vi "Construct.vi"(8 "series":i32(ring)=2 items=["DVP", "AS"], 9 "port":i32=502, 10 "station":u8=1, 11 "ipAddress":string="192.168.1.88") -> (3 "MelsecMcNet out":refnum<class "DeltaTcp.lvclass">)   [LabVIEW 2020, in "HslCommunication.lvlib" / "DeltaTcp.lvclass"]
uses:
  DeltaTcp.lvclass
  DeltaTcp.lvclass/DeltaTcp.ctl
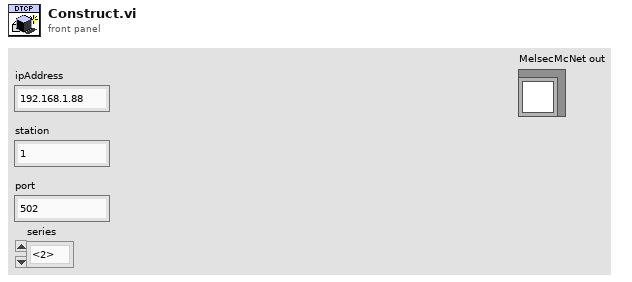
[diagram p1: front panel]
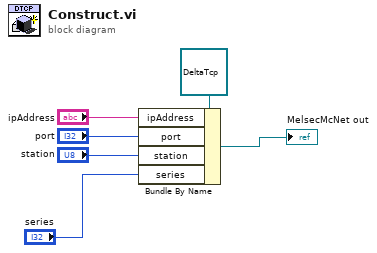
[diagram p0: block diagram]
diagram:
  n1 = Bundle By Name(cluster=refnum<class "DeltaTcp.lvclass"> refnum ("MelsecMcNet in"), "ipAddress"="ipAddress", "port"="port", "station"="station", "series"="series") -> (→"MelsecMcNet out":refnum<class "DeltaTcp.lvclass">)
